vi "setVolume.vi"(8 "error in (no error)":errorcluster, 10 "volume":i32=30, 11 "Tv in":refnum<class "Tv.lvclass">) -> (0 "error out":errorcluster, 3 "Tv out":refnum<class "Tv.lvclass">)   [LabVIEW 2018, in "Tv.lvclass"]
uses:
  Tv.lvclass
  Tv.lvclass/Tv.ctl
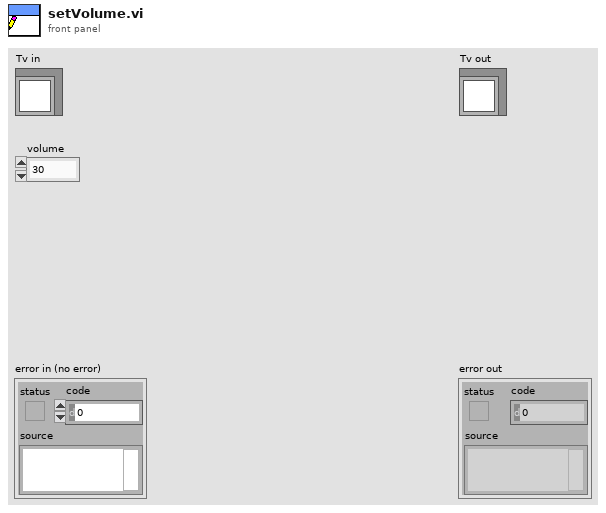
[diagram p1: front panel]
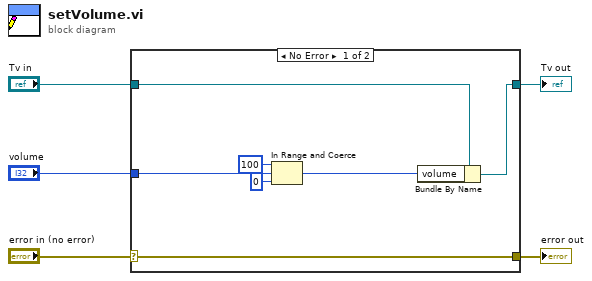
[diagram p0: block diagram]
diagram:
  n1 = case shown="No Error" "error in (no error)" {
    selector: "error in (no error)" -> [w12 w13]
    tunnel: [w12 w13] -> w4
    tunnel: [w10 w14] -> w2
    tunnel: "Tv in" -> [w11 w14]
    tunnel: "volume" -> [w9 _]
    frame No Error {
      n2 = In Range and Coerce(upper limit=100, x=w9, lower limit=0) -> (coerced(x)=w8:i32)  [unwired: 1 out]
      n3 = Bundle By Name(cluster=w11, "volume"=w8) -> (w10:refnum<class "Tv.lvclass">)
    }
    frame Error {
    }
  }
  "error out" <- w4
  "Tv out" <- w2
